vi "显示一组数据不需要输入结果-左上角.vi"(6 "Text Color (black)":u32(colorbox)=16860, 7 "Font, Size & Style":T2={"Desired Font (Application)"=enum."User-specified Font", "[User-specified Font]"={"Font Name"="", "Size"=80, "Strikeout?"=FALSE, "Italic?"=FALSE, "Underline?"=FALSE, "Outline?"=FALSE, "Shadow?"=FALSE, "Bold?"=FALSE, "Rotation Angle"=0.0}, "Horizontal Alignment"=0, "Vertical Alignment"=0} {"Horizontal Alignment" items=["Left", "Center", "Right"]; "Vertical Alignment" items=["Bottom", "Top", "Baseline"]}, 8 "显示坐标 in":cluster{dbl, "Numeric":dbl}[](array[cluster])=[{100.0, "Numeric"=300.0}, {100.0, "Numeric"=400.0}, {100.0, "Numeric"=500.0}, {100.0, "Numeric"=600.0}, {100.0, "Numeric"=700.0}, {100.0, "Numeric"=800.0}, {100.0, "Numeric"=900.0}, {100.0, "Numeric"=1000.0}, {100.0, "Numeric"=1100.0}], 9 "项目名称":string[](array[string]), 10 "待写入数据":dbl[](array[numeric]), 11 "Img输入":T1) -> (3 "Img输出":T1)   [LabVIEW 2014]
uses:
  <vilib>/vision/Image Controls.llb/IMAQ Image.ctl
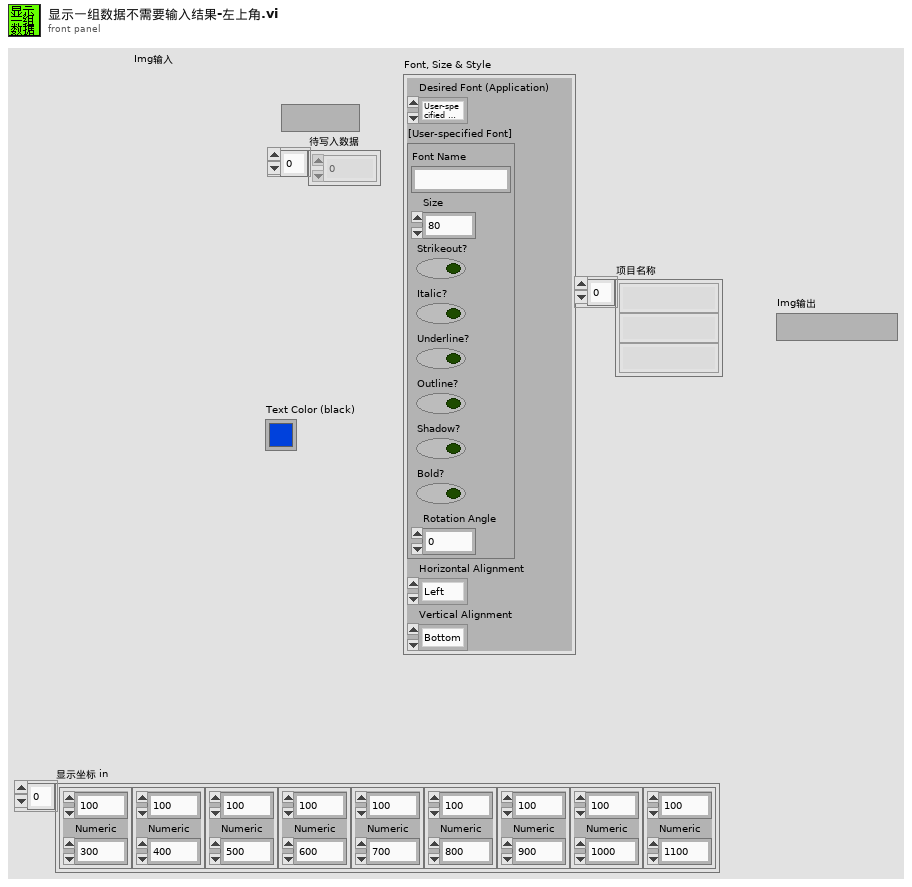
[diagram p1: front panel]
types:
  T1 = typedef "IMAQ Image.ctl" = refnum<image>
  T2 = cluster{"Desired Font (Application)":enum16{"User-specified Font", "Application Font", "System Font", "Dialog Font"}, "[User-specified Font]":cluster{"Font Name":string, "Size":i16, "Strikeout?":bool, "Italic?":bool, "Underline?":bool, "Outline?":bool, "Shadow?":bool, "Bold?":bool, "Rotation Angle":dbl}, "Horizontal Alignment":i16, "Vertical Alignment":i16}
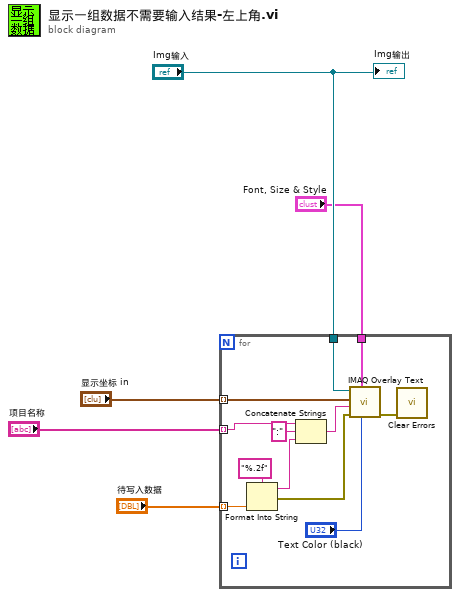
[diagram p0: block diagram]
diagram:
  n1 = for {
    tunnel: "Img输入" -> [w17]
    tunnel: "待写入数据" -> [w16] mode=indexing
    tunnel: "显示坐标 in" -> [w15] mode=indexing
    tunnel: "Font, Size & Style" -> [w14]
    tunnel: "项目名称" -> [w9] mode=indexing
    n2 = Format Into String(format string="%.2f" ("格式字符串"), w16) -> (resulting string=w7:string, error out=w13:errorcluster)  [unwired: 2 in]
    n3 = Concatenate Strings(w9, ":" ("字符串"), w7) -> (w6:string)
    n4 = call "IMAQ Overlay Text"("Text Color (black)"="Text Color (black)", "Font, Size & Style"=w14, "error in (no error)"=w13, "String"=w6, "Origin"=w15, "Image"=w17) -> ("error out"=w12:errorcluster)  [unwired: 4 in, 1 out]
    n5 = call <vilib>:"Clear Errors.vi"("error in (no error)"=w12) -> ()  [unwired: 5 in, 2 out]
  }
  "Img输出" <- "Img输入"
